vi "与副屏通信master.vi"() -> ()   [LabVIEW 2016, in "斯坦道多参数.lvlib"]
uses:
  <vilib>/NI/Modbus Library/API/Wrapper/Create TCP Master.vi
  <vilib>/NI/Modbus Library/API/master/Modbus Master.lvclass
  <vilib>/NI/Modbus Library/API/Wrapper/API Main.lvlib
  <vilib>/ptbypt/NI_PtbyPt.lvlib
panel:
  out "副屏启动命令":u16
  in  "停止 2":bool
  out "read values 2":u16[](array[numeric])
  in  "registers to write 2":u16[](array[numeric])
  out "error out 2":errorcluster caption="error out"
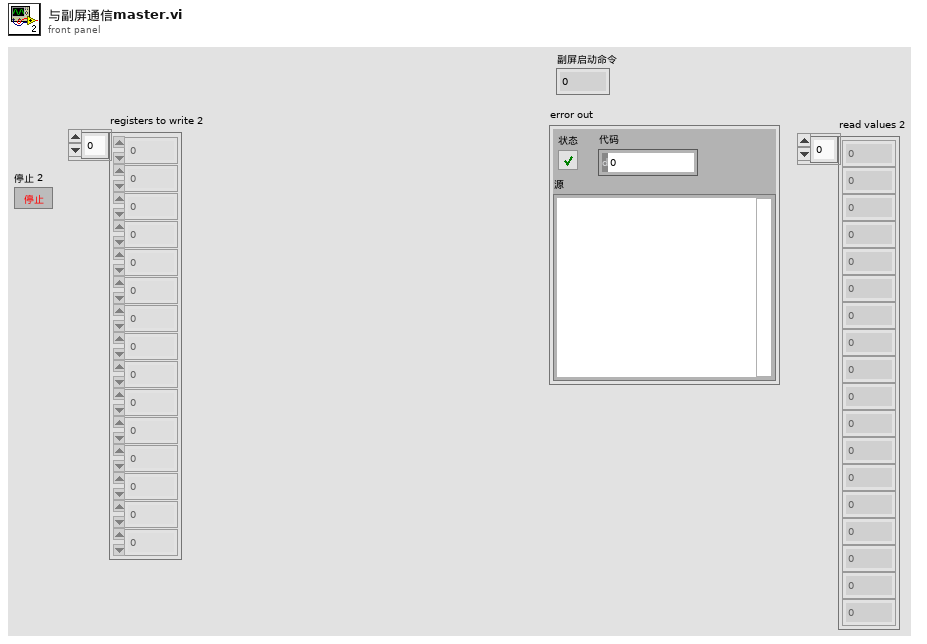
[diagram p1: front panel]
types:
  T1 = cluster{"Boolean array[0]":bool, "Boolean array[1]":bool, "Boolean array[2]":bool, "Boolean array[3]":bool, "Boolean array[4]":bool, "Boolean array[5]":bool, "Boolean array[6]":bool}
  T2 = cluster{"数据保存间隔":dbl, "保存组数":dbl, "水温标样值":dbl, "pH标样值":dbl, "溶解氧标样值":dbl, "电导率标样值":dbl, "浊度标样值":dbl, "pH启用":bool, "溶解氧启用":bool, "电导率启用":bool, "浊度启用":bool}
  T3 = enum32{"Bad", "Idle", "Run top level", "Running"}
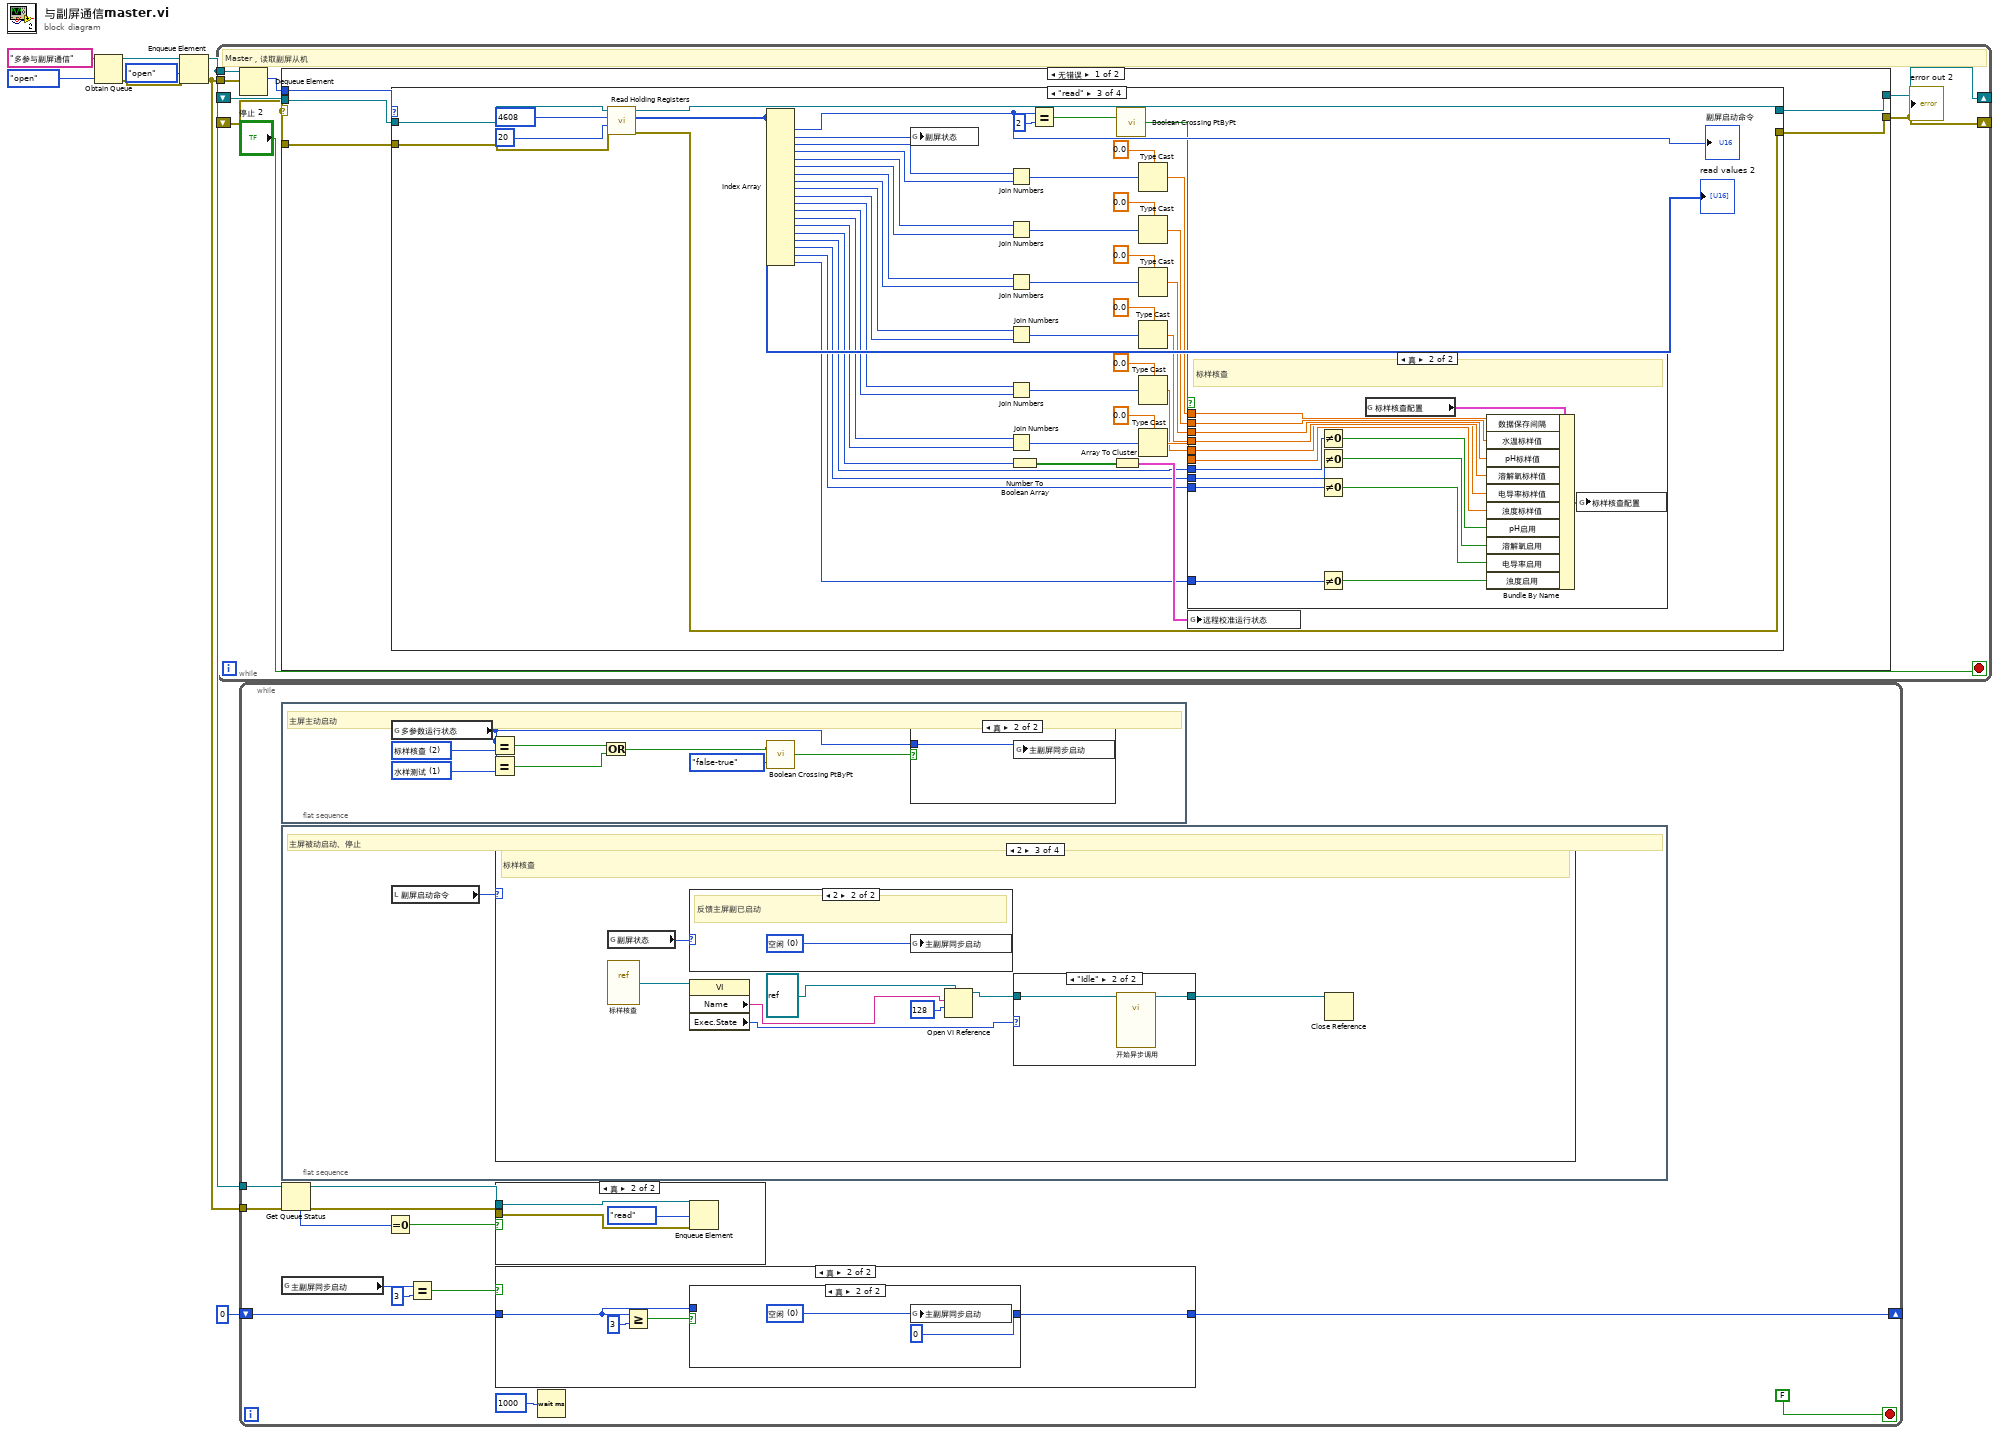
[diagram p0: block diagram]
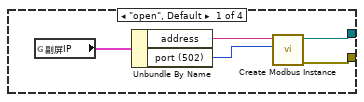
[diagram p2: hidden frame]
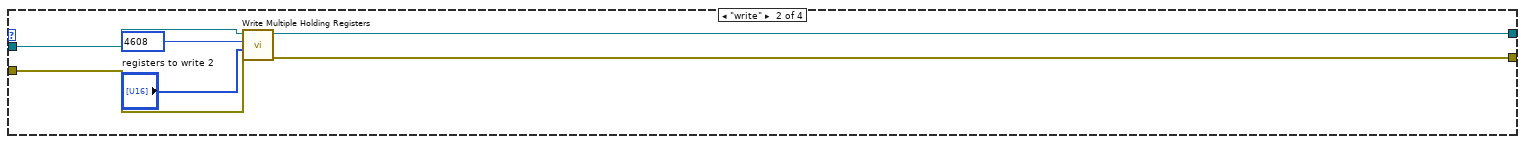
[diagram p3: hidden frame]
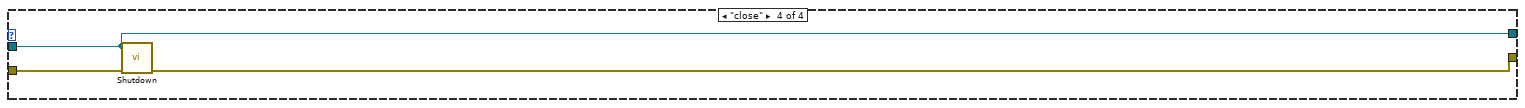
[diagram p5: hidden frame]
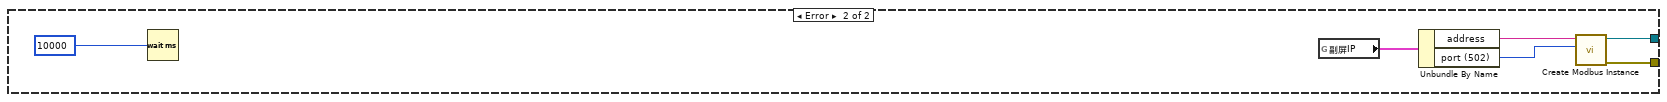
[diagram p6: hidden frame]
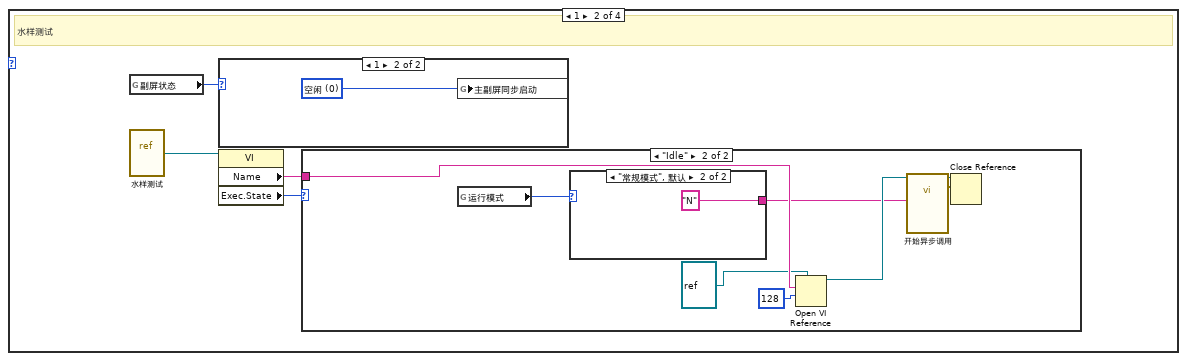
[diagram p8: hidden frame]
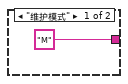
[diagram p11: hidden frame]
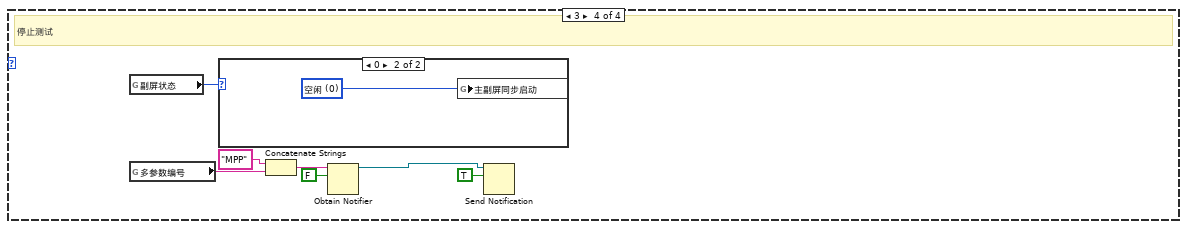
[diagram p14: hidden frame]
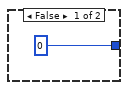
[diagram p16: hidden frame]
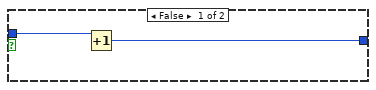
[diagram p17: hidden frame]
diagram:
  n1 = Obtain Queue(name (unnamed)="多参与副屏通信" ("名称（未命名）"), element data type=enum16{"open", "write", "read", "close"}."open") -> (queue out=w5:refnum<queue>, error out=w6:errorcluster)  [unwired: 3 in, 1 out]
  n2 = Enqueue Element(queue=w5, element=enum16{"open", "write", "read", "close"}."open", error in (no error)=w6) -> (queue out=w3:refnum<queue>, error out=w2:errorcluster)  [unwired: 1 in, 1 out]
  n3 = while {
    shift-right: [w13] -> _
    shift-left: _ -> [w15]
    shift-right: [w14] -> _
    shift-left: _ -> [w12]
    tunnel: w3 -> [w11]
    tunnel: w2 -> [w10]
    stop <- "停止 2" stop-if-true
    # "Master，读取副屏从机"
    n4 = Dequeue Element(queue=w11, error in (no error)=w10) -> (element=w9:enum16{"open", "write", "read", "close"})  [unwired: 1 in, 3 out]
    n5 = case shown="无错误" w12 {
      tunnel: w15 -> [w21 _]
      tunnel: w12 -> [w20 _]
      tunnel: [w19 w105] -> w14
      tunnel: [w18 w106] -> w13
      tunnel: w9 -> [w17 _]
      frame No Error {
        n6 = case shown="\"read\"" w17 {
          tunnel: w21 -> [_ w32 w43 w100]
          tunnel: w20 -> [_ w30 w42 w99]
          tunnel: [w25 w27 w40 w98] -> w19
          tunnel: [w26 w28 w41 w100] -> w18
          frame "open", Default {
            n7 = global read "多参数全局变量.vi" "副屏IP"() -> (w24:cluster{"address":string, "port (502)":u16})
            n8 = Unbundle By Name(w24) -> ("address"=w23:string, "port (502)"=w22:u16)
            n9 = call-poly <vilib>:"Create Modbus Instance.vi"("port (502)"=w22, "address"=w23) -> ("error out"=w25:errorcluster, "TCP master instance"=w26:refnum<class "Modbus Master.lvclass">)  [unwired: 8 in]
          }
          frame "write" {
            n10 = call-dynamic "Write Multiple Holding Registers.vi"("error in"=w30, "registers to write"="registers to write 2", "starting address"=u16 4608 ("write starting address"), "Modbus master in"=w32) -> ("error out"=w27:errorcluster, "Modbus master out"=w28:refnum<class "Modbus Master.lvclass">)  [unwired: 6 in]
          }
          frame "read" {
            n11 = call-dynamic "Read Holding Registers.vi"("error in"=w42, "number of inputs"=u16 20 ("read count"), "starting address"=u16 4608 ("write starting address"), "Modbus master in"=w43) -> ("error out"=w40:errorcluster, "register values"=w79:u16[], "Modbus master out"=w41:refnum<class "Modbus Master.lvclass">)  [unwired: 5 in]
            "read values 2" <- w79
            n12 = Index Array(array=w79) -> (element #1=w80:u16, element #2=w81:u16, element #3=w48:u16, element #4=w49:u16, element #5=w55:u16, element #6=w54:u16, element #7=w59:u16, element #8=w58:u16, element #9=w64:u16, element #10=w65:u16, element #11=w72:u16, element #12=w73:u16, element #13=w74:u16, element #14=w75:u16, element #15=w37:u16, element #16=w36:u16, element #17=w35:u16, element #18=w34:u16, element #19=w33:u16)  [unwired: 19 in]
            "副屏启动命令" <- w80
            n13 = global write "多参数全局变量.vi" "副屏状态"(w81) -> ()
            n14 = Join Numbers(hi=w48, lo=w49) -> ((hi.lo)=w47:u32)
            n15 = Join Numbers(hi=w55, lo=w54) -> ((hi.lo)=w52:u32)
            n16 = Join Numbers(hi=w59, lo=w58) -> ((hi.lo)=w57:u32)
            n17 = Join Numbers(hi=w64, lo=w65) -> ((hi.lo)=w62:u32)
            n18 = Join Numbers(hi=w72, lo=w73) -> ((hi.lo)=w67:u32)
            n19 = Join Numbers(hi=w74, lo=w75) -> ((hi.lo)=w69:u32)
            n20 = Number To Boolean Array(number=w37) -> (Boolean array=w39:bool[])
            n21 = Equal?(x=w80, y=u16 2) -> (x = y?=w77:bool)
            n22 = Array To Cluster(array=w39) -> (cluster=w38:T1)
            n23 = call <vilib>:"Boolean Crossing PtByPt.vi"("input"=w77) -> ("crossing"=w78:bool)  [unwired: 2 in]
            n24 = Type Cast(type=sgl 0.0, x=w47) -> (*(type *) &x=w50:sgl)
            n25 = Type Cast(type=sgl 0.0, x=w52) -> (*(type *) &x=w53:sgl)
            n26 = Type Cast(type=sgl 0.0, x=w57) -> (*(type *) &x=w60:sgl)
            n27 = Type Cast(type=sgl 0.0, x=w62) -> (*(type *) &x=w63:sgl)
            n28 = Type Cast(type=sgl 0.0, x=w67) -> (*(type *) &x=w70:sgl)
            n29 = Type Cast(type=sgl 0.0, x=w69) -> (*(type *) &x=w71:sgl)
            n30 = case shown="真" w78 {
              tunnel: w50 -> [_ w95]
              tunnel: w53 -> [_ w94]
              tunnel: w60 -> [_ w93]
              tunnel: w63 -> [_ w92]
              tunnel: w70 -> [_ w91]
              tunnel: w71 -> [_ w90]
              tunnel: w36 -> [_ w89]
              tunnel: w35 -> [_ w85]
              tunnel: w34 -> [_ w87]
              tunnel: w33 -> [_ w86]
              frame False {
              }
              frame True {
                # "标样核查"
                n31 = Not Equal To 0?(x=w89) -> (x != 0?=w88:bool)
                n32 = Not Equal To 0?(x=w85) -> (x != 0?=w84:bool)
                n33 = Not Equal To 0?(x=w87) -> (x != 0?=w83:bool)
                n34 = Not Equal To 0?(x=w86) -> (x != 0?=w82:bool)
                n35 = global read "断电保存变量.vi" "标样核查配置"() -> (w97:T2)
                n36 = Bundle By Name(cluster=w97, "数据保存间隔"=w95, "水温标样值"=w94, "pH标样值"=w93, "溶解氧标样值"=w92, "电导率标样值"=w91, "浊度标样值"=w90, "pH启用"=w88, "溶解氧启用"=w84, "电导率启用"=w83, "浊度启用"=w82) -> (w96:T2)
                n37 = global write "断电保存变量.vi" "标样核查配置"(w96) -> ()
              }
            }
            n38 = global write "多参数全局变量.vi" "远程校准运行状态"(w38) -> ()
          }
          frame "close" {
            n39 = call-dynamic "Shutdown.vi"("error in"=w99, "Modbus master in"=w100) -> ("error out"=w98:errorcluster)  [unwired: 9 in]
          }
        }
      }
      frame Error {
        n40 = Wait (ms)(milliseconds to wait=u32 10000 ("等待时间（毫秒）")) -> ()  [unwired: 1 out]
        n41 = global read "多参数全局变量.vi" "副屏IP"() -> (w103:cluster{"address":string, "port (502)":u16})
        n42 = Unbundle By Name(w103) -> ("address"=w102:string, "port (502)"=w101:u16)
        n43 = call-poly <vilib>:"Create Modbus Instance.vi"("port (502)"=w101, "address"=w102) -> ("error out"=w105:errorcluster, "TCP master instance"=w106:refnum<class "Modbus Master.lvclass">)  [unwired: 8 in]
      }
    }
    "error out 2" <- w14
  }
  n44 = while {
    tunnel: w3 -> [w113]
    tunnel: w2 -> [w112]
    shift-right: [w107] -> _
    shift-left: u32 0 ("等待时间（毫秒）") -> [w108]
    stop <- FALSE stop-if-true
    n45 = flat-sequence {
      frame #0 {
        w167 = u16 2 items=["空闲", "水样测试", "标样核查"] ("多参数运行状态")
        w170 = u16 1 items=["空闲", "水样测试", "标样核查"] ("多参数运行状态")
        # "主屏主动启动"
        n46 = global read "多参数全局变量.vi" "多参数运行状态"() -> (w166:u16)
        n47 = Equal?(x=w166, y=w167) -> (x = y?=w165:bool)
        n48 = Equal?(x=w166, y=w170) -> (x = y?=w171:bool)
        n49 = Or(x=w165, y=w171) -> (x .or. y?=w168:bool)
        n50 = call <vilib>:"Boolean Crossing PtByPt.vi"("direction"=enum16{"either", "false-true", "true-false"}."false-true", "input"=w168) -> ("crossing"=w169:bool)  [unwired: 1 in]
        n51 = case shown="真" w169 {
          tunnel: w166 -> [_ w173]
          frame False {
          }
          frame True {
            n52 = global write "多参数全局变量.vi" "主副屏同步启动"(w173) -> ()
          }
        }
      }
    }
    n53 = flat-sequence {
      frame #0 {
        # "主屏被动启动、停止"
        n54 = local read "副屏启动命令"() -> (w120:u16)
        n55 = case shown="2" w120 {
          frame 0, Default {
          }
          frame 1 {
            # "水样测试"
            n56 = global read "多参数全局变量.vi" "副屏状态"() -> (w121:u16)
            n57 = vi-ref "水样测试.vi"() -> (w124:refnum<vi>)
            n58 = case shown="1" w121 {
              frame 0, Default {
              }
              frame 1 {
                w125 = u16 0 items=["空闲", "水样测试", "标样核查", "停止"] ("主副屏同步启动")
                n59 = global write "多参数全局变量.vi" "主副屏同步启动"(w125) -> ()
              }
            }
            n60 = property class="VI"(reference=w124) -> ("Name"=w122:string, "Exec.State"=w123:T3)  [unwired: 1 in, 2 out]
            n61 = case shown="\"Idle\"" w123 {
              tunnel: w122 -> [_ w130]
              frame "Bad", Default {
              }
              frame "Idle" {
                n62 = global read "多参数全局变量.vi" "运行模式"() -> (w128:enum16{"维护模式", "常规模式", "应急模式", "质控模式"})
                n63 = case shown="\"常规模式\", 默认" w128 {
                  tunnel: ["M" ("数据标记表") "N" ("数据标记表")] -> w127
                  frame "维护模式" {
                  }
                  frame "常规模式", Default {
                  }
                }
                n64 = Open VI Reference(type specifier VI Refnum (for type only)=refnum<vi> refnum, vi path=w130, options=128 ("选项")) -> (vi reference=w131:refnum<vi>)  [unwired: 3 in, 1 out]
                n65 = call-by-ref "开始异步调用"(reference=w131, "数据标记表"=w127) -> (reference out=w132:refnum<vi>, error out=w133:errorcluster)  [unwired: 12 in]
                n66 = Close Reference(reference=w132, error in (no error)=w133) -> ()  [unwired: 1 out]
              }
            }
          }
          frame 2 {
            # "标样核查"
            n67 = global read "多参数全局变量.vi" "副屏状态"() -> (w143:u16)
            n68 = vi-ref "标样核查.vi"() -> (w142:refnum<vi>)
            n69 = case shown="2" w143 {
              frame 0, Default {
              }
              frame 2 {
                w144 = u16 0 items=["空闲", "水样测试", "标样核查", "停止"] ("主副屏同步启动")
                # "反馈主屏副已启动"
                n70 = global write "多参数全局变量.vi" "主副屏同步启动"(w144) -> ()
              }
            }
            n71 = property class="VI"(reference=w142) -> ("Name"=w138:string, "Exec.State"=w140:T3)  [unwired: 1 in, 2 out]
            n72 = Open VI Reference(type specifier VI Refnum (for type only)=refnum<vi> refnum, vi path=w138, options=128 ("选项")) -> (vi reference=w137:refnum<vi>)  [unwired: 3 in, 1 out]
            n73 = case shown="\"Idle\"" w140 {
              tunnel: [w145 w147] -> w141
              tunnel: w137 -> [w145 w146]
              frame "Bad", Default {
              }
              frame "Idle" {
                n74 = call-by-ref "开始异步调用"(reference=w146) -> (reference out=w147:refnum<vi>)  [unwired: 13 in, 1 out]
              }
            }
            n75 = Close Reference(reference=w141) -> ()  [unwired: 1 in, 1 out]
          }
          frame 3 {
            # "停止测试"
            n76 = global read "多参数全局变量.vi" "副屏状态"() -> (w148:u16)
            n77 = global read "多参数全局变量.vi" "多参数编号"() -> (w151:string)
            n78 = case shown="0" w148 {
              frame 1, Default {
              }
              frame 0 {
                w155 = u16 0 items=["空闲", "水样测试", "标样核查", "停止"] ("主副屏同步启动")
                n79 = global write "多参数全局变量.vi" "主副屏同步启动"(w155) -> ()
              }
            }
            n80 = Concatenate Strings("MPP" ("名称（未命名）"), w151) -> (w152:string)
            n81 = Obtain Notifier(name (unnamed)=w152, notification data type=FALSE) -> (notifier out=w149:refnum<notifier>)  [unwired: 2 in, 2 out]
            n82 = Send Notification(notification=TRUE ("通知"), notifier=w149) -> ()  [unwired: 1 in, 2 out]
          }
        }
      }
    }
    n83 = Get Queue Status(queue=w113, error in (no error)=w112) -> (queue out=w115:refnum<queue>, error out=w116:errorcluster, # elements in queue=w114:i32)  [unwired: 1 in, 5 out]
    n84 = global read "多参数全局变量.vi" "主副屏同步启动"() -> (w111:u16)
    n85 = Equal To 0?(x=w114) -> (x = 0?=w117:bool)
    n86 = Equal?(x=w111, y=u16 3) -> (x = y?=w109:bool)
    n87 = case shown="真" w117 {
      tunnel: w115 -> [_ w175]
      tunnel: w116 -> [_ w174]
      frame False {
      }
      frame True {
        n88 = Enqueue Element(queue=w175, element=enum16{"open", "write", "read", "close"}."read", error in (no error)=w174) -> ()  [unwired: 1 in, 3 out]
      }
    }
    n89 = case shown="真" w109 {
      tunnel: w108 -> [_ w159]
      tunnel: [u32 0 w160] -> w107
      frame False {
      }
      frame True {
        n90 = Greater Or Equal?(x=w159, y=u32 3) -> (x >= y?=w157:bool)
        n91 = case shown="真" w157 {
          tunnel: [w162 u32 0] -> w160
          tunnel: w159 -> [w161 _]
          frame False {
            n92 = Increment(x=w161) -> (x+1=w162:u32)
          }
          frame True {
            w164 = u16 0 items=["空闲", "水样测试", "标样核查", "停止"] ("主副屏同步启动")
            n93 = global write "多参数全局变量.vi" "主副屏同步启动"(w164) -> ()
          }
        }
      }
    }
    n94 = Wait (ms)(milliseconds to wait=u32 1000 ("等待时间（毫秒）")) -> ()  [unwired: 1 out]
  }
